vi "Set Item Names in MCListbox.vi"(8 "error in":errorcluster, 9 "Item Names":string[][](array[string]), 10 "Label":string, 11 "Class in":refnum<class>) -> (0 "error out":errorcluster, 3 "Class out":refnum<class>)   [LabVIEW 2023, in "Label-Driven UI.lvlib"]
uses:
  Label-Driven UI.lvlib
  28948a29-962f-49c8-956d-8245adfcffa2.vi
  28948a29-962f-49c8-956d-8245adfcffa2.vi/8fe3da84-711b-404a-8a89-ddc030b01c8b.vi
  Get VI Ref.vi
  Include Control Ref in Tab.vi
  Append Label to Error.vi
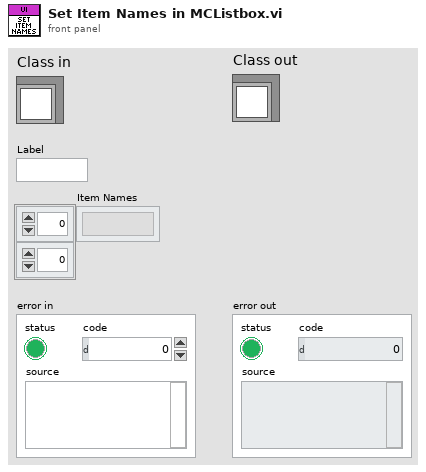
[diagram p1: front panel]
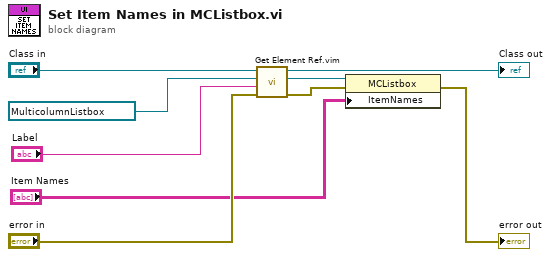
[diagram p0: block diagram]
diagram:
  n1 = call "Get Element Ref.vim"("error in"="error in", "Label"="Label", "Ref Type"=refnum<vi> refnum, "Class in"="Class in") -> ("error out"=w3:errorcluster, "Element Ref"=w4:refnum<vi>, "Class out"=→"Class out":refnum<class>)  [unwired: 5 in]
  n2 = property class="MCListbox"(reference=w4, error in=w3, "ItemNames"="Item Names") -> (error out=→"error out":errorcluster)  [unwired: 1 out]
